vi "Old Main.vi"() -> ()   [LabVIEW 2020]
doc: "Retrieves average CPU temp, if available. No warranty, use it at your own risk.\n\n© Aitor Solar, 2019.\nContact: aitor.solar@gmail.com"
uses:
  <vilib>/Platform/TimedLoop/XDataNode/timing_clust.ctl
  <vilib>/Platform/TimedLoop/XDataNode/nitl_modes.ctl
  <vilib>/Platform/TimedLoop/XDataNode/wakeup.ctl
  <vilib>/platform/TimedLoop/XDataNode/XDataNode.xnode
  <vilib>/Platform/TimedLoop/XDataNode/XDNodeRunTimeDep.lvlib
panel:
  in  "Read System Temps":bool
  out "Output Filename":path
  in  "Create New File":bool=TRUE
  out "Waveform Chart":dbl[](graph)
  in  "stop":bool
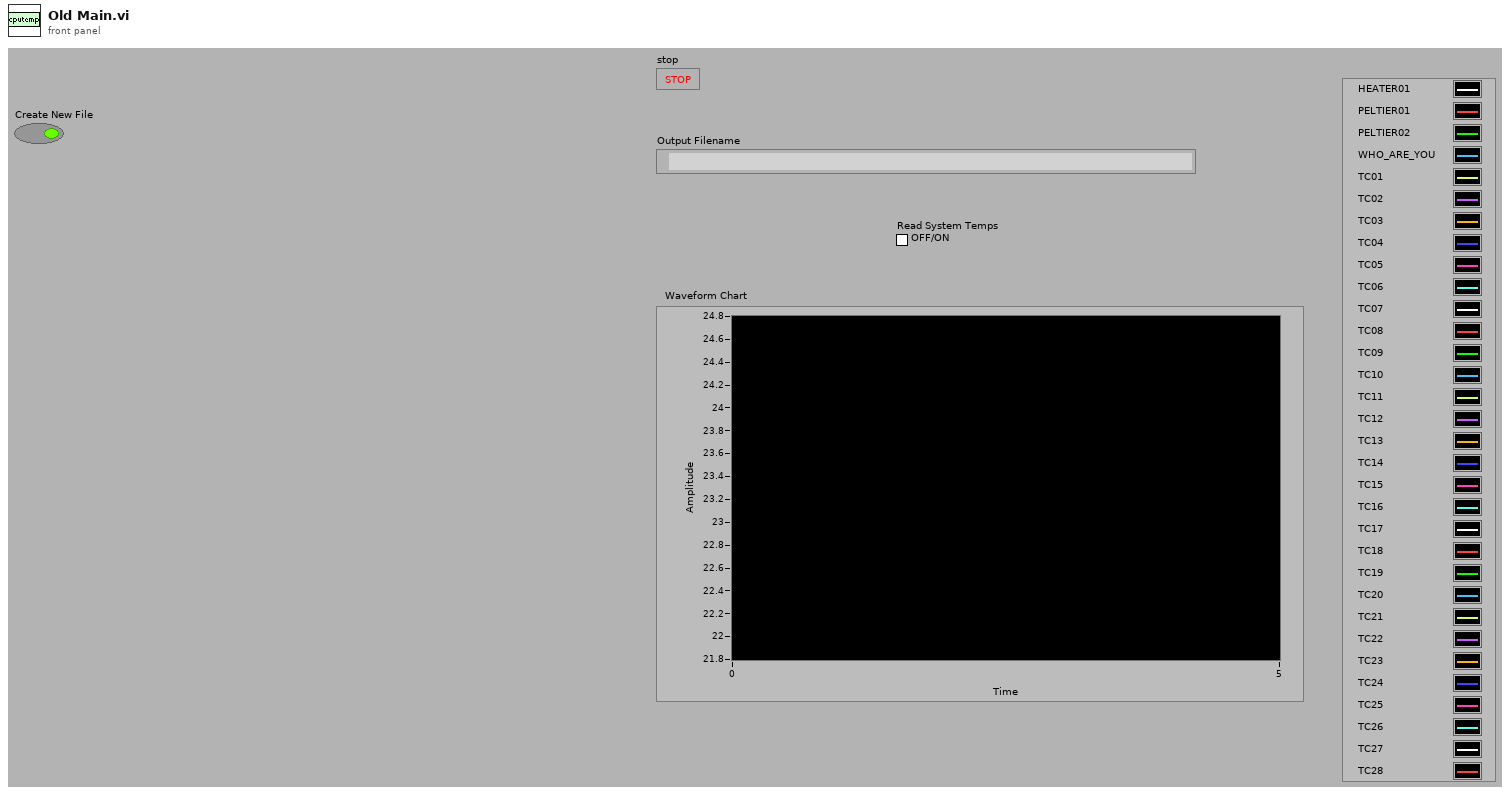
[diagram p1: front panel]
types:
  T1 = typedef "XDNodeRunTimeDep.lvlib/timing_clust.ctl" = cluster{"Expected End [f-1]":u64, "Actual End [f-1]":u64, "Finished Late? [f-1]":bool, "Expected End [i-1]":u64, "Actual End [i-1]":u64, "Finished Late? [i-1]":bool, "Expected Start [i]":u64, "Actual Start [i]":u64, "Expected Start [f]":u64, "Actual Start [f]":u64, "Source Name":string, "Structure Name":string, "Period":i64, "Deadline":i64, "Offset":i64, "Start":i64, "Priority":i32, "Timeout":i32, "Mode":T2, "Wakeup Reason":T3, "Error":errorcluster, "Source Type":string, "Secondary Source Type":string, "Global End Time":u64, "Global Start Time":u64, "Frame Duration":u64, "Iteration Duration":u64, "Assigned CPU":i32, "I/O Scan Engine Mode":u32}
  T2 = typedef "XDNodeRunTimeDep.lvlib/nitl_modes.ctl" = enum32{"No Change", "Process missed periods, maintain original phase", "Discard missed periods, maintain original phase", "Process missed periods, ignore original phase", "Discard missed periods, ignore original phase"}
  T3 = typedef "XDNodeRunTimeDep.lvlib/wakeup.ctl" = enum32{"Normal", "Aborted", "Asynchronous wakeup", "Timing source error", "Timed loop error", "Timeout"}
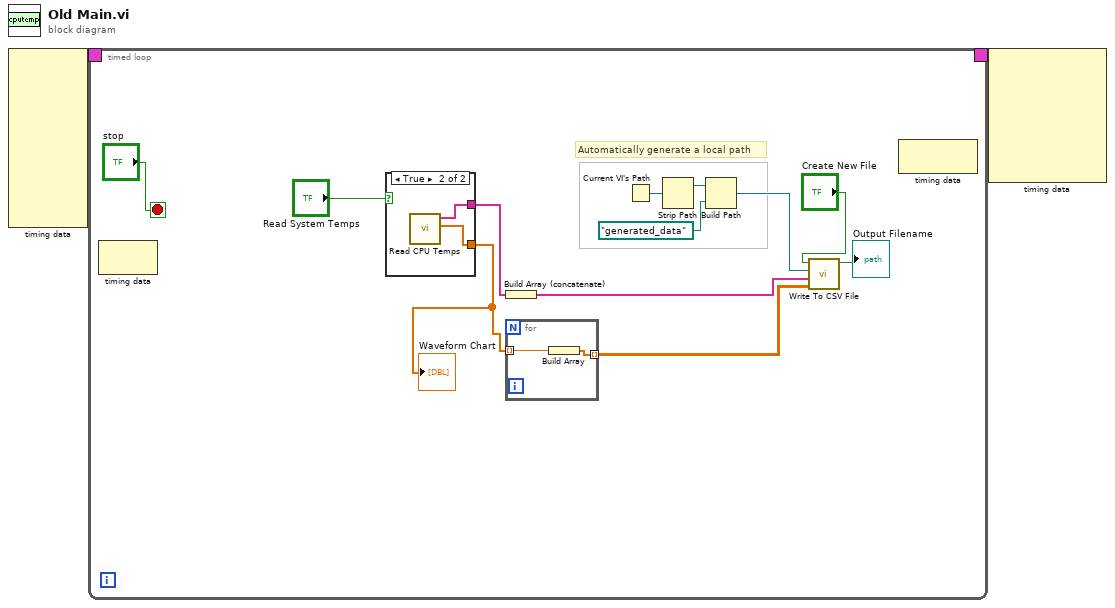
[diagram p0: block diagram]
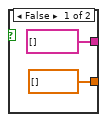
[diagram p2: hidden frame]
diagram:
  n1 = node-c288() -> (w2:T1)  [unwired: 10 in]
  n2 = timed-loop {
    timing: w2 -> [_]
    timing-out: [_] -> w1
    stop <- "stop" stop-if-true
    # "Automatically generate a local path"
    n3 = node-c288() -> ()  [unwired: 1 in, 1 out]
    n4 = case shown="True" "Read System Temps" {
      tunnel: [string[] [] ("Names") w18] -> w9
      tunnel: [dbl[] [] ("Termperatures") w17] -> w3
      frame False {
      }
      frame True {
        n5 = call "Read CPU Temps.vi"() -> ("Termperatures"=w17:dbl[], "Names"=w18:string[])  [unwired: 9 in, 1 out]
      }
    }
    "Waveform Chart" <- w3
    n6 = Build Array (concatenate)(w9) -> (w12:string[])
    n7 = for {
      tunnel: w3 -> [w20] mode=indexing
      tunnel: [w19] -> w11 mode=indexing
      n8 = Build Array(w20) -> (w19:dbl[])
    }
    n9 = Current VI's Path() -> (path=w7:path)
    n10 = Strip Path(path=w7) -> (stripped path=w6:path)  [unwired: 1 out]
    n11 = Build Path(base path=w6, name or relative path=path "generated_data") -> (appended path=w4:path)
    n12 = call "Write To CSV File.vi"("Values"=w11, "Names"=w12, "Output Directory"=w4, "Create New File"="Create New File") -> ("Output Filename"=→"Output Filename":path)  [unwired: 7 in]
    n13 = node-c288() -> ()  [unwired: 1 in, 1 out]
  }
  n14 = node-c288(w1) -> ()  [unwired: 7 out]
